vi "CRYCalculate User Equation.vi"(10 "No.VI":i32, 11 "User equation cluster In":T2 {"Results axis" items=["x", "y", "z"]; "Input axis" items=["x", "y", "z"]; "Custom unit results array"."dB ref" format="%.2f"; "Custom unit input array"."dB ref" format="%.2f"}) -> (1 "Result Curves":T1[](array[typedef]) {"Z data" items=["dB", "Lin"]; "X data" items=["dB", "Lin"]; "Y data" items=["dB", "Lin"]; "Z dB ref" format="%.1f"; "Z axis" items=["Log", "Lin"]; "X dB ref" format="%.1f"; "X axis" items=["Log", "Lin"]; "Y axis" items=["Log", "Lin"]; "Y dB ref" format="%.1f"; "Curve"."z" format="%.2f"; "Curve"."y" format="%.2f"; "Curve"."x" format="%.2f"}, 2 "Types":enum16{"Curves", "Values", "Results", "WFM"}[](array[ring]), 3 "User equation cluster Out":T2 {"Results axis" items=["x", "y", "z"]; "Input axis" items=["x", "y", "z"]; "Custom unit results array"."dB ref" format="%.2f"; "Custom unit input array"."dB ref" format="%.2f"})   [LabVIEW 2013]
uses:
  Typedef Control/CRYUser Equation Cluster.ctl
  Typedef Control/CRYData Cluster.ctl
  CRYProject/CRYProject Editor Global.vi
  <vilib>/gmath/NI_Gmath.lvlib
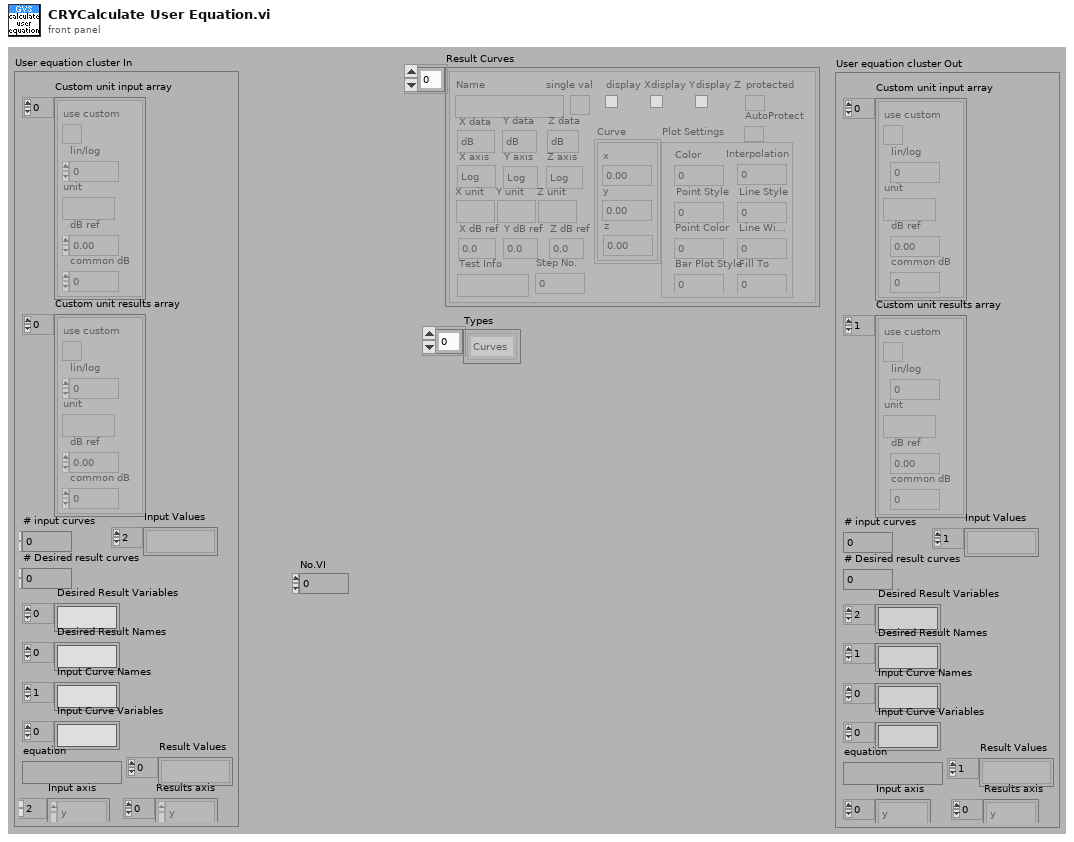
[diagram p1: front panel]
types:
  T1 = typedef "CRYData Cluster.ctl" = cluster{"Name":string, "Curve":cluster{"x":dbl, "y":dbl, "z":dbl}[], "X data":u16, "Y data":u16, "Z data":u16, "X axis":u16, "Y axis":u16, "Z axis":u16, "X unit":string, "Y unit":string, "Z unit":string, "X dB ref":dbl, "Y dB ref":dbl, "Z dB ref":dbl, "single val":bool, "protected":bool, "display X":bool, "display Y":bool, "display Z":bool, "Test Info":string, "Step No.":i32, "Plot Settings":cluster{"Color":u32, "Interpolation":u8, "Point Style":u8, "Line Style":u8, "Point Color":u32, "Line Width":u8, "Bar Plot Style":u8, "Fill To":i16}, "AutoProtect":bool}
  T2 = typedef "CRYUser Equation Cluster.ctl" = cluster{"Custom unit input array":cluster{"use custom":bool, "lin/log":u16, "unit":string, "dB ref":dbl, "common dB":u16}[], "Custom unit results array ":cluster{"use custom":bool, "lin/log":u16, "unit":string, "dB ref":dbl, "common dB":u16}[], "Desired Result Variables":string[], "Desired Result Names":string[], "Input Curve Names":string[], "Input Curve Variables":string[], "equation":string, "Input axis":u16[], "Results axis":u16[], "# input curves":i32, "# Desired result curves ":i32, "Input Values":string[], "Result Values":string[]}
  T3 = typedef "CRYData Cluster Array.ctl" = T1[]
  T4 = cluster{"use custom":bool, "lin/log":u16, "unit":string, "dB ref":dbl, "common dB":u16}[]
  T5 = enum16{"OK", "Yes", "YesNo", "YesNoCancel", "ReplaceAppend"}
  T6 = cluster{"use custom":bool, "lin/log":u16, "unit":string, "dB ref":dbl, "common dB":u16}
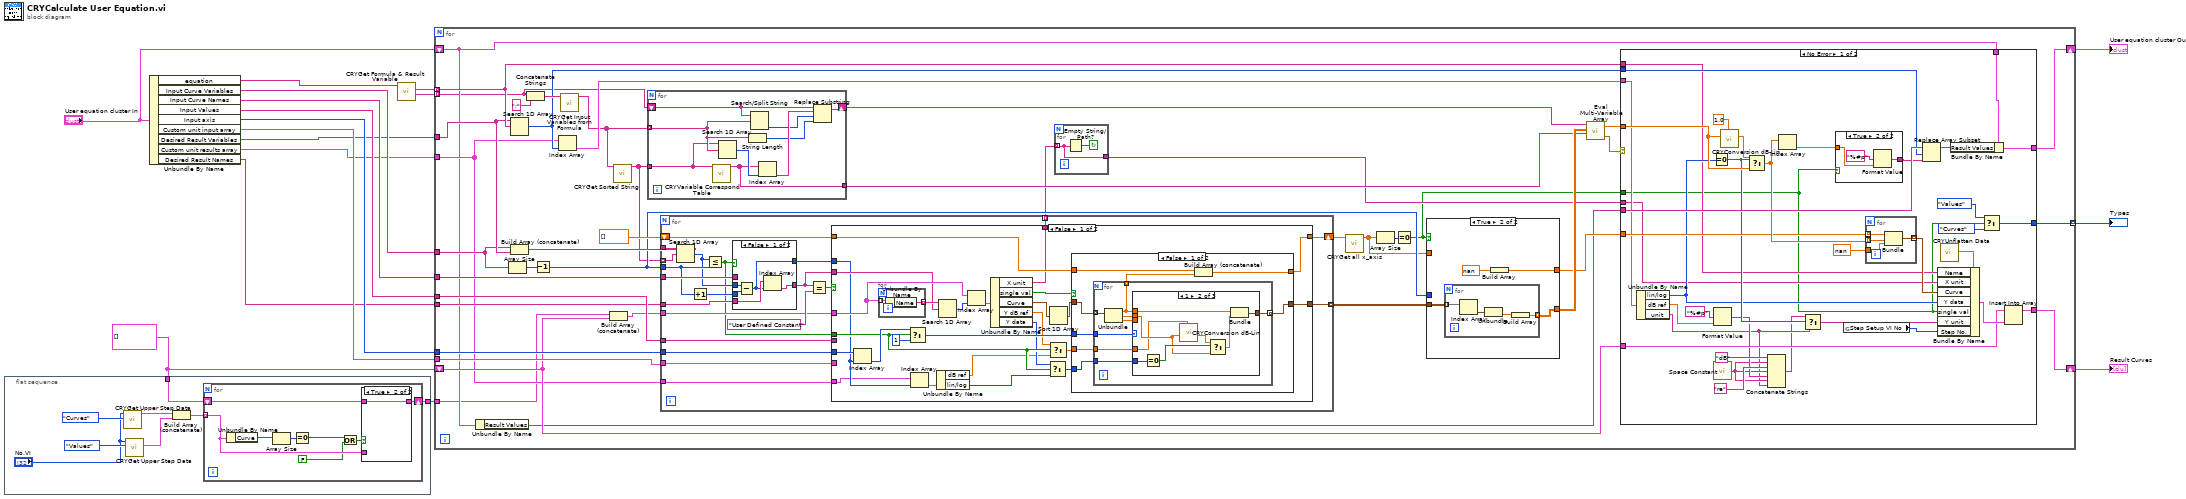
[diagram p0: block diagram]
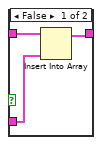
[diagram p2: hidden frame]
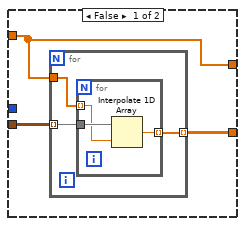
[diagram p3: hidden frame]
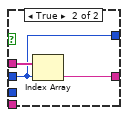
[diagram p4: hidden frame]
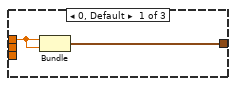
[diagram p5: hidden frame]
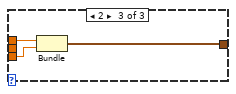
[diagram p6: hidden frame]
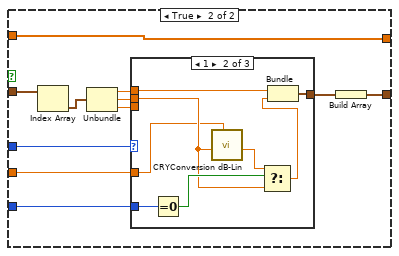
[diagram p7: hidden frame]
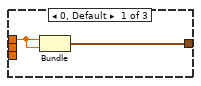
[diagram p8: hidden frame]
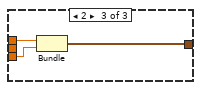
[diagram p9: hidden frame]
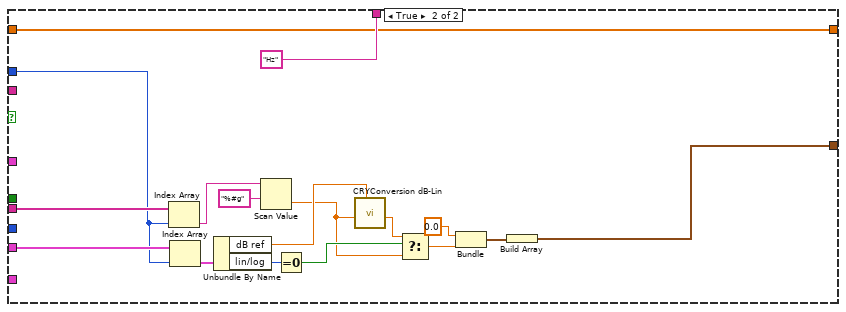
[diagram p10: hidden frame]
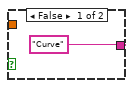
[diagram p11: hidden frame]
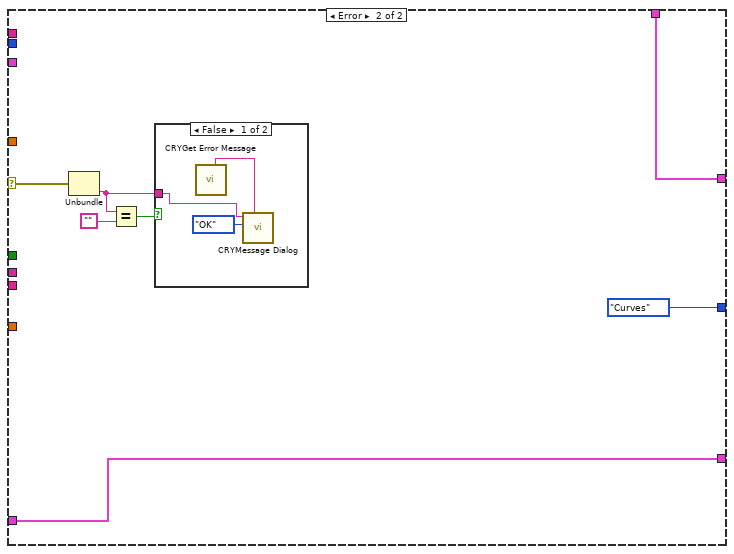
[diagram p12: hidden frame]
diagram:
  w3 = T1[] [] ("Result Curves")
  n1 = flat-sequence {
    tunnel: w3 -> [w25]
    tunnel: [w23] -> w2
    frame #0 {
      n2 = call "CRYGet Upper Step Data.vi"("Type In"=enum16{"Curves", "Values", "Results", "WFM"}."Curves", "No.VI"="No.VI") -> ("Curve array"=w20:T3)  [unwired: 9 out]
      n3 = call "CRYGet Upper Step Data.vi"("Type In"=enum16{"Curves", "Values", "Results", "WFM"}."Values", "No.VI"="No.VI") -> ("Value array"=w19:T3)  [unwired: 9 out]
      n4 = Build Array (concatenate)(w20, w19) -> (w24:T3)
      n5 = for {
        shift-right: [w30] -> w23
        shift-left: w25 -> [w31]
        tunnel: w24 -> [w29] mode=indexing
        n6 = Unbundle By Name(w29) -> ("Curve"=w33:cluster{"x":dbl, "y":dbl, "z":dbl}[])
        n7 = Array Size(array=w33) -> (size(s)=w32:i32)
        n8 = Equal To 0?(x=w32) -> (x = 0?=w27:bool)
        n9 = Or(x=w27, y=FALSE ("t")) -> (x .or. y?=w28:bool)
        n10 = case shown="True" w28 {
          tunnel: w31 -> [w36 w37]
          tunnel: [w35 w37] -> w30
          tunnel: w29 -> [w34 _]
          frame False {
            n11 = Insert Into Array(array=w36, new element=w34) -> (w35:T1[])  [unwired: 1 in]
          }
          frame True {
          }
        }
      }
    }
  }
  n12 = Unbundle By Name("User equation cluster In") -> ("equation"=w14:string, "Input Curve Variables"=w8:string[], "Input Curve Names"=w12:string[], "Input Values"=w11:string[], "Input axis"=w10:u16[], "Custom unit input array"=w9:T4, "Desired Result Variables"=w7:string[], "Custom unit results array"=w6:T4, "Desired Result Names"=w1:string[])
  n13 = call "CRYGet Formula & Result Variable.vi"("String"=w14) -> ("Formula Out"=w15:string[], "Result Variable"=w13:string[])  [unwired: 8 in, 1 out]
  n14 = for {
    tunnel: w15 -> [w51] mode=indexing
    tunnel: w13 -> [w70] mode=indexing
    tunnel: w8 -> [w58]
    tunnel: w12 -> [w76]
    tunnel: w11 -> [w75]
    tunnel: w10 -> [w74]
    tunnel: w9 -> [w71]
    tunnel: w7 -> [w60]
    tunnel: w6 -> [w54]
    shift-right: [w69] -> w16
    shift-left: "User equation cluster In" -> [w53]
    shift-right: [w67] -> w5
    shift-left: w3 -> [w68]
    tunnel: [w66] -> w4 mode=indexing
    tunnel: w1 -> [w55]
    tunnel: w2 -> [w42]
    n15 = Unbundle By Name(w53) -> ("Result Values"=w52:string[])
    n16 = Array Size(array=w58) -> (size(s)=w57:i32)
    n17 = Search 1D Array(1D array=w60, element=w70) -> (index of element=w62:i32)  [unwired: 1 in]
    n18 = Build Array (concatenate)(w58, w60) -> (w59:string[])
    n19 = Concatenate Strings(w51, ";" ("string")) -> (w77:string)
    n20 = Decrement(x=w57) -> (x-1=w56:i32)
    n21 = Index Array(array=w54, index=w62) -> (element=w61:T6)
    n22 = call "CRYGet Input Variables from Formula.vi"("Formula string"=w77) -> ("Variables Out"=w50:string[])  [unwired: 10 in]
    n23 = Build Array (concatenate)(w42, w68) -> (w41:T1[])
    n24 = call "CRYGet Sorted String.vi"("Variables In"=w50) -> ("Variables Out"=w43:string[])  [unwired: 10 in]
    n25 = for {
      tunnel: w50 -> [w228] mode=indexing
      shift-right: [w227] -> w49
      shift-left: w51 -> [w229]
      tunnel: [w226] -> w48
      tunnel: w43 -> [w225]
      n26 = call "CRYVariable Correspond Table.vi"("Variables In"=w225) -> ("New Variables"=w226:string[])  [unwired: 9 in, 1 out]
      n27 = Search 1D Array(1D array=w225, element=w228) -> (index of element=w232:i32)  [unwired: 1 in]
      n28 = String Length(string=w228) -> (length=w231:i32)
      n29 = Search/Split String(string=w229, search string/char (-)=w228) -> (offset of match=w230:i32)  [unwired: 1 in, 2 out]
      n30 = Index Array(array=w226, index=w232) -> (element=w233:string)
      n31 = Replace Substring(2:w231, 3:w230, 4:w233, 5:w229) -> (1:w227:string)  [unwired: 1 out]
    }
    n32 = for {
      tunnel: w43 -> [w118] mode=indexing
      tunnel: w59 -> [w117]
      tunnel: w76 -> [w116]
      tunnel: w41 -> [w112]
      shift-right: [w110] -> w47
      shift-left: dbl[] [] -> [w111]
      tunnel: [w109] -> w40 mode=indexing
      tunnel: w56 -> [w108]
      tunnel: w55 -> [w106]
      tunnel: w75 -> [w104]
      tunnel: w71 -> [w103]
      tunnel: w74 -> [w102]
      tunnel: w54 -> [w100]
      tunnel: [w98] -> w44 mode=indexing
      n33 = Search 1D Array(1D array=w117, element=w118) -> (index of element=w105:i32)  [unwired: 1 in]
      n34 = Increment(x=w108) -> (x+1=w107:i32)
      n35 = Less Or Equal?(x=w105, y=w108) -> (x <= y?=w101:bool)
      n36 = case shown="False" w101 {
        tunnel: w116 -> [_ w126]
        tunnel: [w120 w125] -> w113
        tunnel: w105 -> [w123 w124]
        tunnel: w107 -> [w122 _]
        tunnel: w106 -> [w121 _]
        tunnel: [w119 w124] -> w99
        frame False {
          n37 = Subtract(x=w123, y=w122) -> (x-y=w119:i32)
          n38 = Index Array(array=w121, index=w119) -> (element=w120:string)
        }
        frame True {
          n39 = Index Array(array=w126, index=w124) -> (element=w125:string)
        }
      }
      n40 = Equal?(x=w113, y="User Defined Constant") -> (x = y?=w114:bool)
      n41 = case shown="False" w114 {
        tunnel: w113 -> [w149 _]
        tunnel: w112 -> [w150 _]
        tunnel: w111 -> [w146 w223]
        tunnel: [w145 w223] -> w110
        tunnel: [w144 "Hz" ("String")] -> w109
        tunnel: w99 -> [w134 w220]
        tunnel: w104 -> [_ w222]
        tunnel: w103 -> [_ w221]
        tunnel: w102 -> [w143 _]
        tunnel: w101 -> [w138 _]
        tunnel: [w139 w208] -> w98
        tunnel: w100 -> [w133 _]
        frame False {
          n42 = Index Array(array=w143, index=w134) -> (element=w142:u16)
          n43 = for {
            tunnel: w150 -> [w207] mode=indexing
            tunnel: [w206] -> w152 mode=indexing
            n44 = Unbundle By Name(w207) -> ("Name"=w206:string)
          }
          n45 = Select(t=w142, s=w138, f=u16 1) -> (s? t:f=w140:u16)
          n46 = Index Array(array=w133, index=w134) -> (element=w135:T6)
          n47 = Unbundle By Name(w135) -> ("dB ref"=w132:dbl, "lin/log"=w131:u16)
          n48 = Search 1D Array(1D array=w152, element=w149) -> (index of element=w151:i32)  [unwired: 1 in]
          n49 = Index Array(array=w150, index=w151) -> (element=w148:T1)
          n50 = Unbundle By Name(w148) -> ("X unit"=w144:string, "single val"=w147:bool, "Curve"=w128:cluster{"x":dbl, "y":dbl, "z":dbl}[], "Y dB ref"=w137:dbl, "Y data"=w136:u16)
          n51 = Select(t=w136, s=w138, f=w131) -> (s? t:f=w129:u16)
          n52 = Select(t=w137, s=w138, f=w132) -> (s? t:f=w130:dbl)
          n53 = Sort 1D Array(array=w128) -> (sorted array=w127:cluster{"x":dbl, "y":dbl, "z":dbl}[])
          n54 = case shown="False" w147 {
            tunnel: w127 -> [w158 w191]
            tunnel: w146 -> [w160 w192]
            tunnel: [w159 w192] -> w145
            tunnel: w140 -> [w157 w190]
            tunnel: [w156 w184] -> w139
            tunnel: w130 -> [w154 w182]
            tunnel: w129 -> [w153 w183]
            frame False {
              n55 = for {
                tunnel: w158 -> [w168] mode=indexing
                tunnel: w157 -> [w167]
                tunnel: [w164] -> w156 mode=indexing
                tunnel: [w163] -> w155 mode=indexing
                tunnel: w154 -> [w162]
                tunnel: w153 -> [w161]
                n56 = Unbundle(w168) -> ("x"=w163:dbl, "y"=w166:dbl, "z"=w165:dbl)
                n57 = case shown="1" w167 {
                  tunnel: w163 -> [w170 w178 w181]
                  tunnel: w166 -> [_ w173 _]
                  tunnel: w165 -> [_ _ w180]
                  tunnel: [w169 w177 w179] -> w164
                  tunnel: w162 -> [_ w172 _]
                  tunnel: w161 -> [_ w175 _]
                  frame 0, Default {
                    n58 = Bundle("x"=w170, "x"=w170) -> (w169:cluster{"x":dbl, "x":dbl})  [unwired: 1 in]
                  }
                  frame 1 {
                    n59 = Equal To 0?(x=w175) -> (x = 0?=w174:bool)
                    n60 = call "CRYConversion dB-Lin.vi"("dB ref."=w172, "Log In"=w173) -> ("Lin Out"=w176:dbl)  [unwired: 4 in, 3 out]
                    n61 = Select(t=w176, s=w174, f=w173) -> (s? t:f=w171:dbl)
                    n62 = Bundle("x"=w178, "y"=w171) -> (w177:cluster{"x":dbl, "y":dbl})  [unwired: 1 in]
                  }
                  frame 2 {
                    n63 = Bundle("x"=w181, "z"=w180) -> (w179:cluster{"x":dbl, "z":dbl})  [unwired: 1 in]
                  }
                }
              }
              n64 = Build Array (concatenate)(w160, w155) -> (w159:dbl[])
            }
            frame True {
              n65 = Index Array(array=w191) -> (element=w188:cluster{"x":dbl, "y":dbl, "z":dbl})  [unwired: 1 in]
              n66 = Unbundle(w188) -> ("x"=w189:dbl, "y"=w187:dbl, "z"=w186:dbl)
              n67 = case shown="1" w190 {
                tunnel: w189 -> [w194 w202 w205]
                tunnel: w187 -> [_ w197 _]
                tunnel: w186 -> [_ _ w204]
                tunnel: [w193 w201 w203] -> w185
                tunnel: w183 -> [_ w200 _]
                tunnel: w182 -> [_ w196 _]
                frame 0, Default {
                  n68 = Bundle("x"=w194, "x"=w194) -> (w193:cluster{"x":dbl, "x":dbl})  [unwired: 1 in]
                }
                frame 1 {
                  n69 = Equal To 0?(x=w200) -> (x = 0?=w198:bool)
                  n70 = call "CRYConversion dB-Lin.vi"("dB ref."=w196, "Log In"=w197) -> ("Lin Out"=w199:dbl)  [unwired: 4 in, 3 out]
                  n71 = Select(t=w199, s=w198, f=w197) -> (s? t:f=w195:dbl)
                  n72 = Bundle("x"=w202, "y"=w195) -> (w201:cluster{"x":dbl, "y":dbl})  [unwired: 1 in]
                }
                frame 2 {
                  n73 = Bundle("x"=w205, "z"=w204) -> (w203:cluster{"x":dbl, "z":dbl})  [unwired: 1 in]
                }
              }
              n74 = Build Array(w185) -> (w184:cluster{"x":dbl, "z":dbl}[])
            }
          }
        }
        frame True {
          n75 = Index Array(array=w222, index=w220) -> (element=w216:string)
          n76 = Index Array(array=w221, index=w220) -> (element=w218:T6)
          n77 = Unbundle By Name(w218) -> ("dB ref"=w213:dbl, "lin/log"=w219:u16)
          n78 = Scan Value(string=w216, format string="%#g") -> (value=w212:dbl)  [unwired: 1 in, 1 out]
          n79 = Equal To 0?(x=w219) -> (x = 0?=w214:bool)
          n80 = call "CRYConversion dB-Lin.vi"("dB ref."=w213, "Log In"=w212) -> ("Lin Out"=w215:dbl)  [unwired: 4 in, 3 out]
          n81 = Select(t=w215, s=w214, f=w212) -> (s? t:f=w211:dbl)
          n82 = Bundle("s? t:f"=0.0, "Lin Out"=w211) -> (w209:cluster{"s? t:f":dbl, "Lin Out":dbl})  [unwired: 1 in]
          n83 = Build Array(w209) -> (w208:cluster{"s? t:f":dbl, "Lin Out":dbl}[])
        }
      }
    }
    n84 = for {
      tunnel: w40 -> [w79] mode=indexing
      tunnel: [w79] -> w39
      stop <- w80 continue-if-true
      n85 = Empty String/Path?(string/path=w79) -> (empty?=w80:bool)
    }
    n86 = call "CRYGet all x_axis.vi"("x_Array in"=w47) -> ("X_axis out"=w45:dbl[])  [unwired: 10 in]
    n87 = Array Size(array=w45) -> (size(s)=w46:i32)
    n88 = Equal To 0?(x=w46) -> (x = 0?=w38:bool)
    n89 = case shown="True" w38 {
      tunnel: [w81 w90] -> w64
      tunnel: [w82 w92] -> w63
      tunnel: w45 -> [w82 _]
      tunnel: w56 -> [_ _]
      tunnel: w44 -> [w83 w91]
      frame False {
        n90 = for {
          tunnel: w83 -> [w85] mode=indexing
          tunnel: w82 -> [w86]
          tunnel: [w84] -> w81 mode=indexing
          n91 = for {
            tunnel: w86 -> [w88] mode=indexing
            tunnel: w85 -> [w89]
            tunnel: [w87] -> w84 mode=indexing
            n92 = Interpolate 1D Array(1:w88, 2:w89) -> (0:w87:dbl)
          }
        }
      }
      frame True {
        n93 = for {
          tunnel: w91 -> [w97] mode=indexing
          tunnel: [w94] -> w90 mode=indexing
          n94 = Index Array(array=w97) -> (element=w96:cluster{"s? t:f":dbl, "Lin Out":dbl})  [unwired: 1 in]
          n95 = Unbundle(w96) -> ("Lin Out"=w95:dbl)  [unwired: 1 out]
          n96 = Build Array(w95) -> (w94:dbl[])
        }
        n97 = Build Array(nan ("value")) -> (w92:dbl[])
      }
    }
    n98 = call <vilib>:"Eval Multi-Variable Array.vi"("Variables"=w48, "X Values"=w64, "formula"=w49) -> ("error out"=w72:errorcluster, "Y Values"=w73:dbl[])  [unwired: 1 in]
    n99 = case shown="No Error" w72 {
      selector: w72 -> [_ w285]
      tunnel: w73 -> [w269 _]
      tunnel: w70 -> [w236 _]
      tunnel: w52 -> [w265 _]
      tunnel: w53 -> [w266 w281]
      tunnel: [w262 w281] -> w69
      tunnel: w68 -> [w255 w280]
      tunnel: [w254 w280] -> w67
      tunnel: [w251 enum16{"Curves", "Values", "Results", "WFM"}."Curves" ("f")] -> w66
      tunnel: w63 -> [w250 _]
      tunnel: w62 -> [w249 _]
      tunnel: w61 -> [w247 _]
      tunnel: w39 -> [w235 _]
      tunnel: w38 -> [w234 _]
      frame No Error {
        n100 = Unbundle By Name(w247) -> ("lin/log"=w246:u16, "dB ref"=w244:dbl, "unit"=w239:string)
        n101 = Equal To 0?(x=w246) -> (x = 0?=w248:bool)
        n102 = Format Value(format string="%#p", value (0)=w244) -> (output string=w241:string)  [unwired: 1 in]
        n103 = call <vilib>:"Space Constant.vi"() -> ("String"=w240:string)
        n104 = call "CRYConversion dB-Lin.vi"("dB ref."=1.0, "Lin In array"=w269) -> ("Log Out array"=w268:dbl[])  [unwired: 4 in, 3 out]
        n105 = Select(t=w268, s=w248, f=w269) -> (s? t:f=w260:dbl[])
        n106 = Concatenate Strings("dB" ("string"), w240, "re" ("string"), w240, w241, w240, w239) -> (w238:string)
        n107 = Index Array(array=w260) -> (element=w267:dbl)  [unwired: 1 in]
        n108 = Select(t=w238, s=w248, f=w239) -> (s? t:f=w237:string)
        n109 = case shown="True" w234 {
          tunnel: w267 -> [_ w278]
          tunnel: ["Curve" ("output string") w276] -> w264
          frame False {
          }
          frame True {
            n110 = Format Value(format string="%#p", value (0)=w278) -> (output string=w276:string)  [unwired: 1 in]
          }
        }
        n111 = global read "CRYProject Editor Global.vi" "Step Setup VI No"() -> (w257:i32)
        n112 = for {
          tunnel: w260 -> [w274] mode=indexing
          tunnel: nan -> [w273]
          tunnel: [w272] -> w258 mode=indexing
          tunnel: w250 -> [w271] mode=indexing
          n113 = Bundle("value"=w271, "result"=w274, w273) -> (w272:cluster{"value":dbl, "result":dbl, dbl})  [unwired: 1 in]
        }
        n114 = Replace Array Subset(array=w265, new element=w264, index=w249) -> (w263:string[])
        n115 = call "CRYUnflatten Data.vi"() -> ("Datum"=w261:T1)  [unwired: 9 in, 2 out]
        n116 = Bundle By Name(cluster=w261, "Name"=w236, "X unit"=w235, "Curve"=w258, "Y data"=w246, "single val"=w234, "Y unit"=w237, "Step No."=w257) -> (w256:T1)
        n117 = Bundle By Name(cluster=w266, "Result Values"=w263) -> (w262:T2)
        n118 = Select(t=enum16{"Curves", "Values", "Results", "WFM"}."Values" ("Type out"), s=w234, f=enum16{"Curves", "Values", "Results", "WFM"}."Curves") -> (s? t:f=w251:enum16{"Curves", "Values", "Results", "WFM"})
        n119 = Insert Into Array(array=w255, new element=w256) -> (w254:T1[])  [unwired: 1 in]
      }
      frame Error {
        n120 = Unbundle(w285) -> ("source"=w282:string)  [unwired: 2 out]
        n121 = Equal?(x=w282, y="") -> (x = y?=w283:bool)
        n122 = case shown="False" w283 {
          tunnel: w282 -> [w286 _]
          frame False {
            n123 = call "CRYGet Error Message.vi"() -> ("Window Title"=w287:string)  [unwired: 6 in, 5 out]
            n124 = call "CRYMessage Dialog.vi"("Window Title"=w287, "YesNoCancel"=T5."OK", "Message Content"=w286) -> ()  [unwired: 7 in, 2 out]
          }
          frame True {
          }
        }
      }
    }
  }
  "User equation cluster Out" <- w16
  "Result Curves" <- w5
  "Types" <- w4
